vi "Get Selected XNET Channels.vi"(6 "Add Info?":bool, 8 "error in (no error)":errorcluster, 9 "Node Ptr":u64 format="%.0x", 10 "XNET Cluster":refnum<k21>, 11 "Tree In":refnum<vi>) -> (0 "error out":errorcluster, 2 "XNET Signal Names":refnum<k21>[](array[refnum]), 3 "Tree Out":refnum<vi>)   [LabVIEW 2025, in "Protection and Counter Addon System Explorer.lvlib"]
uses:
  Protection and Counter Addon System Explorer.lvlib
  <vilib>/NI VeriStand/Custom Device API/Custom Device API.lvlib
panel:
  # "OUTPUTS"
  # "INPUTS"
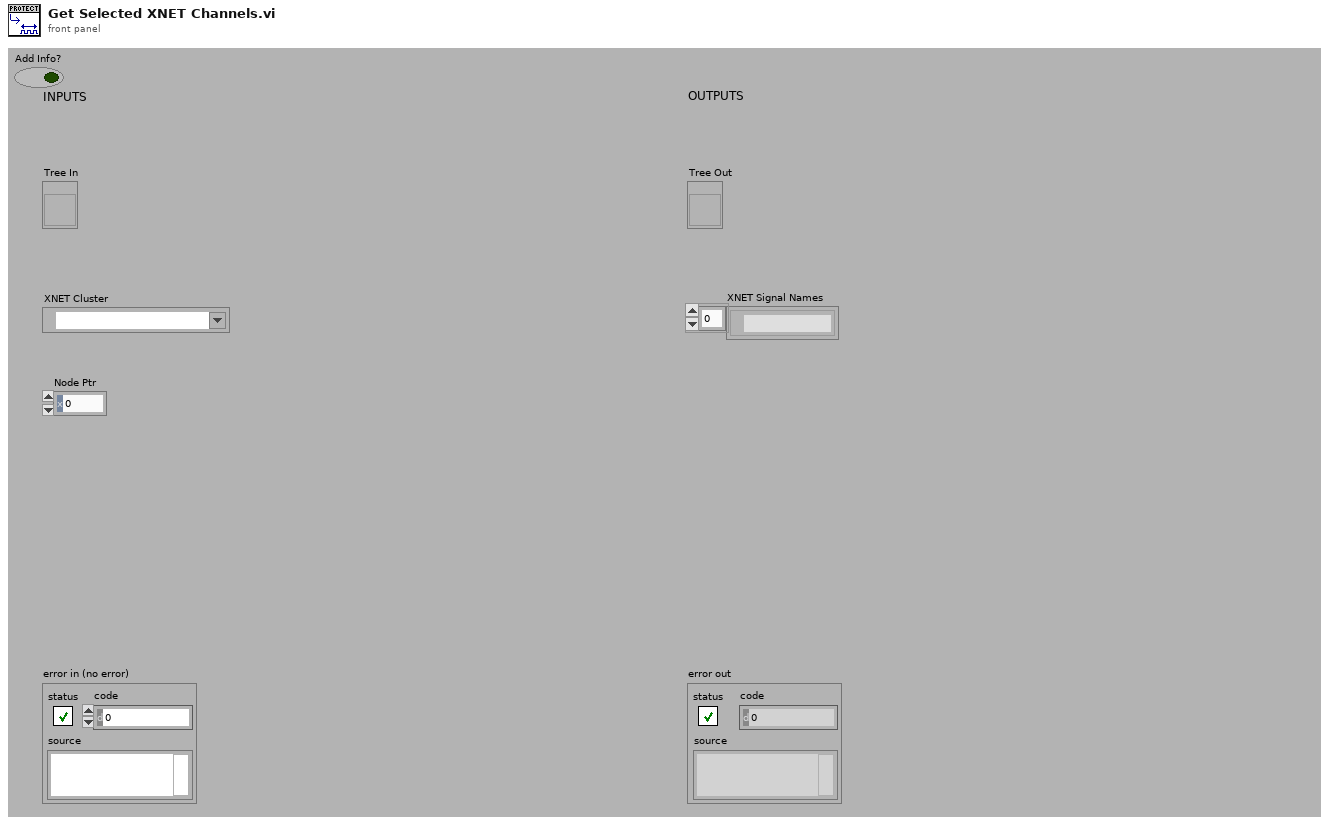
[diagram p1: front panel]
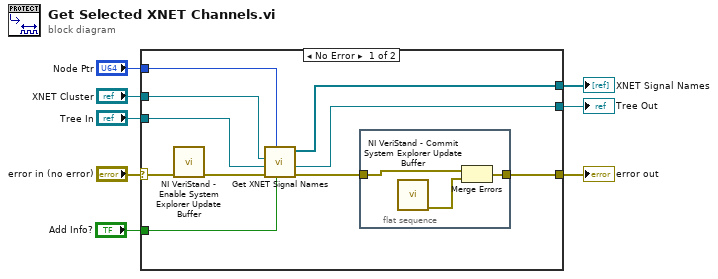
[diagram p0: block diagram]
diagram:
  n1 = case shown="No Error" "error in (no error)" {
    selector: "error in (no error)" -> [w15 w23]
    tunnel: [w13 w23] -> w7
    tunnel: "XNET Cluster" -> [w9 _]
    tunnel: [w17 _] -> w5
    tunnel: "Tree In" -> [w16 w22]
    tunnel: [w18 w22] -> w3
    tunnel: "Node Ptr" -> [w11 _]
    tunnel: "Add Info?" -> [w12 _]
    frame No Error {
      n2 = call <vilib>:"NI VeriStand - Enable System Explorer Update Buffer.vi"("error in (no error)"=w15) -> ("error out"=w10:errorcluster)  [unwired: 10 in]
      n3 = call "Get XNET Signal Names.vi"("Add Info?"=w12, "Parent Ref in"=w11, "error in"=w10, "Tree In"=w16, "XNET Cluster"=w9) -> ("error out"=w14:errorcluster, "Tree Out"=w18:refnum<vi>, "XNET Signal Names"=w17:refnum<k21>[])  [unwired: 4 in]
      n4 = flat-sequence {
        tunnel: w14 -> [w20]
        tunnel: [w19] -> w13
        frame #0 {
          n5 = call <vilib>:"NI VeriStand - Commit System Explorer Update Buffer.vi"() -> ("error out"=w21:errorcluster)  [unwired: 11 in]
          n6 = Merge Errors(w20, w21) -> (w19:errorcluster)
        }
      }
    }
    frame Error {
    }
  }
  "error out" <- w7
  "XNET Signal Names" <- w5
  "Tree Out" <- w3
